vi "test SSL Client Invalid Hostname.vi"(8 "error in (no error)":errorcluster, 11 "TestCase in":refnum<class "test SSL Client.lvclass">) -> (0 "error out":errorcluster, 3 "TestCase out":refnum<class "test SSL Client.lvclass">)   [LabVIEW 2013, in "test SSL Client.lvclass"]
uses:
  test SSL Client.lvclass
  SSL_Lib/SSL/SSL_Mode.ctl
  <vilib>/Utility/error.llb/DialogType.ctl
  suite SSL Client/suite SSL Client/SSL Context.vi
  <vilib>/addons/_JKI Toolkits/VI Tester/TestCase.llb/TestCase.lvclass
  SSL_Lib/BIO/BIO.lvclass
  SSL_Lib/SSL-Context/SSL-Context.lvclass
  SSL_Lib/SSL/SSL.lvclass
  suite SSL Client/suite SSL Client/suite SSL Client.lvclass
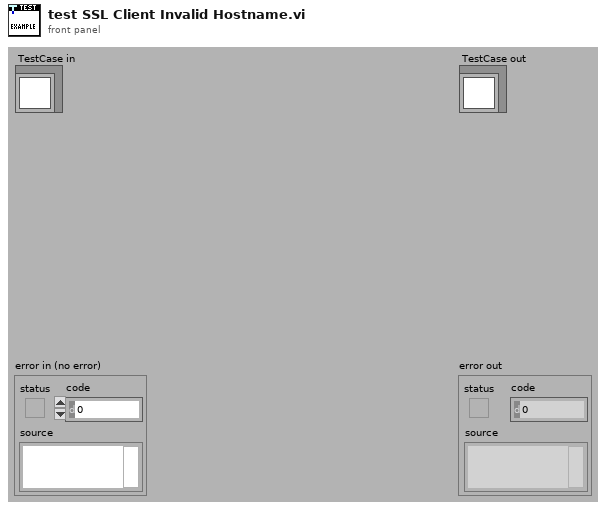
[diagram p1: front panel]
types:
  T1 = typedef "SSL_Lib.lvlib/SSL.lvclass/SSL_Mode.ctl" = i32
  T2 = typedef "DialogType.ctl" = u16
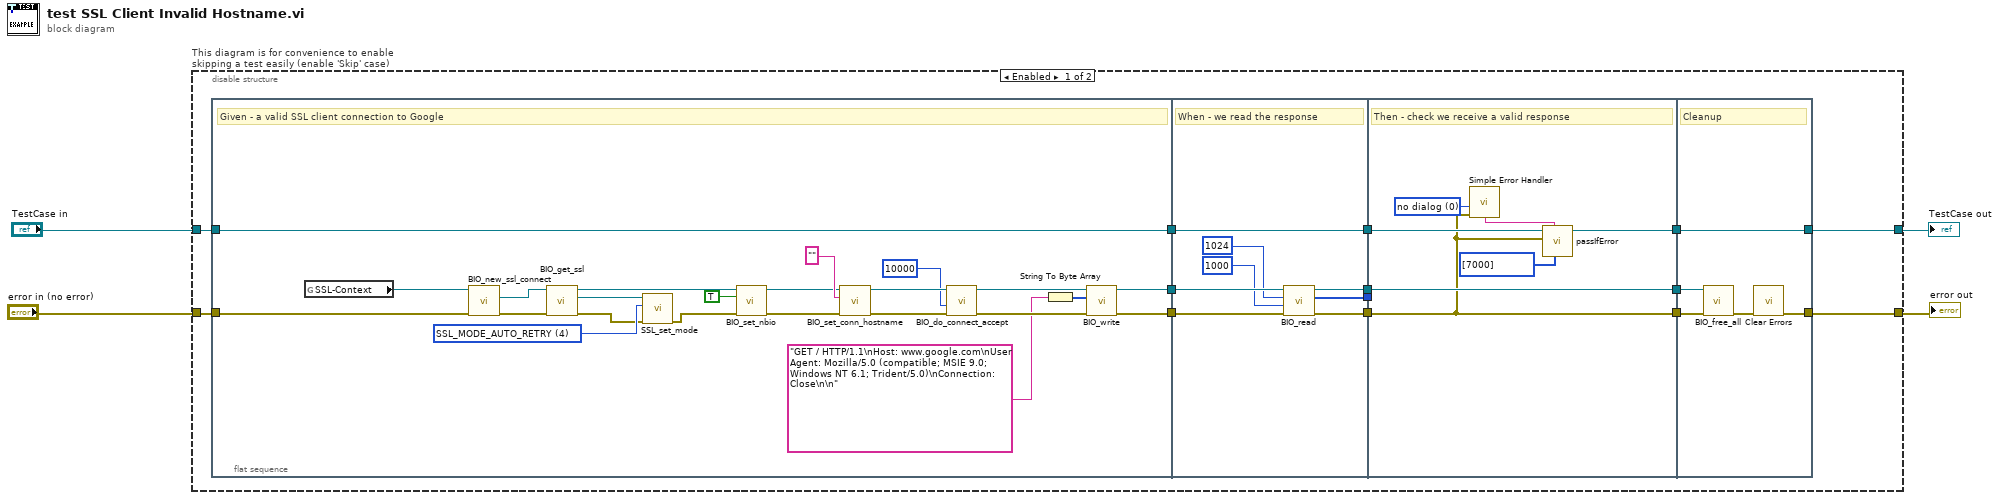
[diagram p0: block diagram]
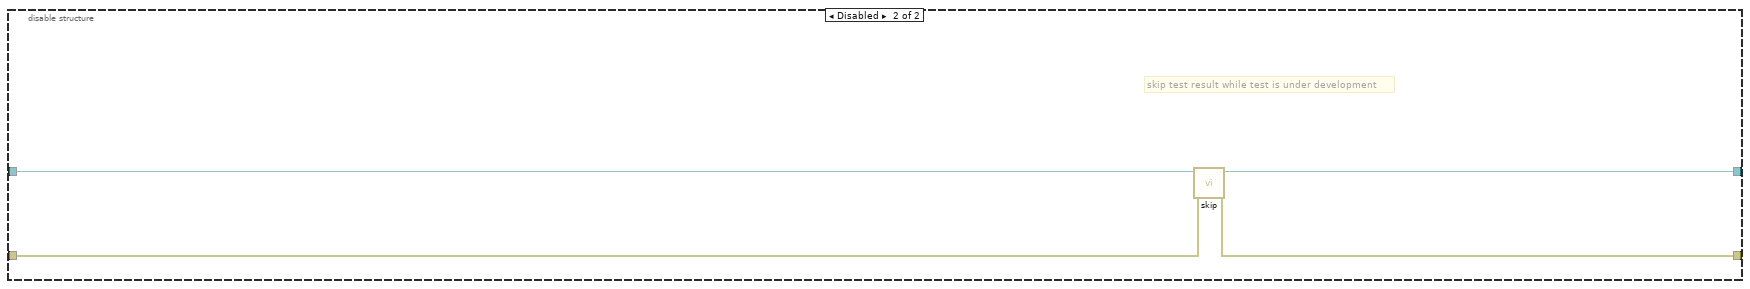
[diagram p2: hidden frame]
diagram:
  n1 = disable-structure "This diagram is for convenience to enable skipping a test easily (enable 'Skip' case)" shown="Enabled" {
    disable-tunnel: "TestCase in" -> [w13 w65]
    disable-tunnel: [w12 w63] -> w1
    disable-tunnel: [w11 w64] -> w3
    disable-tunnel: "error in (no error)" -> [w14 w62]
    frame Enabled {
      n2 = flat-sequence {
        tunnel: w14 -> [w29]
        tunnel: w13 -> [w28]
        tunnel: [w28] -> w18
        tunnel: [w37] -> w10
        tunnel: [w36] -> w9
        tunnel: [w49] -> w17
        tunnel: [w46] -> w16
        tunnel: w18 -> [w49]
        tunnel: w10 -> [w48]
        tunnel: w9 -> [w47]
        tunnel: [w45] -> w8
        tunnel: [w44] -> w7
        tunnel: [w55] -> w15
        tunnel: w17 -> [w56]
        tunnel: w16 -> [w50]
        tunnel: w8 -> [_]
        tunnel: w7 -> [w51]
        tunnel: [w51] -> w6
        tunnel: [w50] -> w5
        tunnel: [w57] -> w11
        tunnel: [w61] -> w12
        tunnel: w15 -> [w61]
        tunnel: w6 -> [w58]
        tunnel: w5 -> [w60]
        frame #0 {
          w31 = T1 4 items=["None"=0, "SSL_MODE_ENABLE_PARTIAL_WRITE"=1, "SSL_MODE_ACCEPT_MOVING_WRITE_BUFFER"=2, "SSL_MODE_AUTO_RETRY"=4, "SSL_MODE_RELEASE_BUFFERS"=16, "SSL_MODE_SEND_FALLBACK_SCSV"=128] ("Mode")
          # "Given - a valid SSL client connection to Google"
          n3 = global read "SSL Context.vi" "SSL-Context"() -> (w27:refnum<class "SSL-Context.lvclass">)
          n4 = call "BIO_new_ssl_connect.vi"("error in (no error)"=w29, "SSL-Context in"=w27) -> ("error out"=w33:errorcluster, "BIO out"=w34:refnum<class "BIO.lvclass">)  [unwired: 7 in, 1 out]
          n5 = call "BIO_get_ssl.vi"("error in (no error)"=w33, "BIO in"=w34) -> ("error out"=w30:errorcluster, "SSL out"=w32:refnum<class "SSL.lvclass">, "BIO out"=w24:refnum<class "BIO.lvclass">)  [unwired: 7 in]
          n6 = call "SSL_set_mode.vi"("error in (no error)"=w30, "Mode"=w31, "SSL in"=w32) -> ("error out"=w25:errorcluster)  [unwired: 7 in, 1 out]
          n7 = call "BIO_set_nbio.vi"("error in (no error)"=w25, "Non-Blocking?"=TRUE, "BIO in"=w24) -> ("error out"=w22:errorcluster, "BIO out"=w23:refnum<class "BIO.lvclass">)  [unwired: 7 in]
          n8 = call "BIO_set_conn_hostname.vi"("error in (no error)"=w22, "Hostname"="", "BIO in"=w23) -> ("error out"=w40:errorcluster, "BIO out"=w35:refnum<class "BIO.lvclass">)  [unwired: 7 in]
          n9 = call "BIO_do_connect_accept.vi"("error in (no error)"=w40, "Timeout (10000ms)"=u32 10000, "BIO in"=w35) -> ("error out"=w39:errorcluster, "BIO out"=w38:refnum<class "BIO.lvclass">)  [unwired: 7 in]
          n10 = String To Byte Array(string="GET / HTTP/1.1\nHost: www.google.com\nUser Agent: Mozilla/5.0 (compatible; MSIE 9.0; Windows NT 6.1; Trident/5.0)\nConnection: Close\n\n" ("String to write")) -> (unsigned byte array=w19:u8[])
          n11 = call "BIO_write.vi"("error in (no error)"=w39, "Bytes to write"=w19, "BIO in"=w38) -> ("error out"=w37:errorcluster, "BIO out"=w36:refnum<class "BIO.lvclass">)  [unwired: 6 in, 1 out]
        }
        frame #1 {
          # "When - we read the response"
          n12 = call "BIO_read.vi"("error in (no error)"=w48, "Timeout (10000ms)"=u32 1000, "bytes to read"=1024, "BIO in"=w47) -> ("error out"=w46:errorcluster, "Bytes read"=w45:u8[], "BIO out"=w44:refnum<class "BIO.lvclass">)  [unwired: 5 in]
        }
        frame #2 {
          w52 = T2 0 items=["no dialog", "OK message", "continue or stop message", "OK message + warnings", "continue/stop + warnings"] ("type of dialog (OK msg:1)")
          # "Then - check we receive a valid response"
          n13 = call <vilib>:"Simple Error Handler.vi"("type of dialog (OK msg:1)"=w52, "error in (no error)"=w50) -> ("message"=w53:string)  [unwired: 3 in, 4 out]
          n14 = call-dynamic "passIfError.vi"("passing error codes (default = any error code)"=i32[] [7000], "custom report message (\"\")"=w53, "error"=w50, "TestCase in"=w56) -> ("TestCase out"=w55:refnum<class "test SSL Client.lvclass">)  [unwired: 6 in, 1 out]
        }
        frame #3 {
          # "Cleanup"
          n15 = call "BIO_free_all.vi"("error in (no error)"=w60, "BIO in"=w58) -> ("error out"=w59:errorcluster)  [unwired: 9 in]
          n16 = call <vilib>:"Clear Errors.vi"("error in (no error)"=w59) -> ("error out"=w57:errorcluster)  [unwired: 6 in]
        }
      }
    }
    frame Disabled {
      # "skip test result while test is under development"
      n17 = call <vilib>:"skip.vi"("error in (no error)"=w62, "TestCase in"=w65) -> ("error out"=w64:errorcluster, "TestCase out"=w63:refnum<class "test SSL Client.lvclass">)  [unwired: 8 in]
    }
  }
  "error out" <- w3
  "TestCase out" <- w1
